vi "ShooterHoodPositionControl.vi"(0 "ShooterHoodMotorControlDevRef":T1={"DeviceStatus"={"status"=FALSE, "code"=0, "source"=""}, "Type"=enum."PWM", "PWM"={"PWM Channel"=enum."PWM 1", "DeadBand"={"Name"="", "maxPositivePwm"=0, "minPositivePwm"=0, "centerPwm"=0, "maxNegativePwm"=0, "minNegativePwm"=0, "angularRange"=0}}, "CAN"={"Device Number"=0, "SetOutput VI Ref"=variant(enum8{"Percent VBus", "Current", "Speed", "Position", "Voltage"} enum."Percent VBus"), "GetOutput VI Ref"=variant(refnum<k1> refnum), "Enable VI Ref"=variant(dbl 12.0), "Disable VI Ref"=variant(enum8{"Percent VBus", "Speed", "Position", "Slave", "Unchanged / Invalid", "Voltage Compensation", "Current", "Motion Profile"} enum."Percent VBus"), "Data"=variant}, "Invert"=FALSE, "DIO PWM"={"PWM \"Enable\" Channel"=enum."Invalid", "DIOChannel"=enum."Invalid", "PWM Rate"=0.0}}, 1 "Activate Auto":bool, 2 "MotorConfig":T6={"CAN Address"=0, "Invert"=FALSE, "InvertSensor"=FALSE, "Unit Conversion Factor"=0.0, "Brake Mode"=enum."Override to Brake", "Reverse Limt Switch Mode"=enum."Disabled", "Forward Limt Swith Mode"=enum."Disabled", "PWM Channel"=enum."Invalid", "Motor Controller Type"=enum."Talon SRX", "Peak Current (A)"=0, "Continuous Current (A)"=0, "Peak Duration (ms)"=0, "Current Limit Enable"=FALSE}, 3 "SetPoint(Deg)":dbl, 4 "ManualControl":dbl min=0.0 max=1.0) -> (5 "Manual?":bool, 6 "Current Position (Deg)":dbl)   [LabVIEW 2019]
uses:
  <vilib>/Rock Robotics/WPI/ThirdParty/Phoenix-LabVIEW/Motor Controller/Controls/CTRE_Phoenix_MotorControl_ControlMode.ctl
  ArgosLib/Config/ConfigComponents/TypeDefs/Config_PIDParams.ctl
  ArgosLib/ArgosLib.lvlib
  <vilib>/Rock Robotics/WPI/ThirdParty/Phoenix-LabVIEW/Motor Controller/Get/CTRE_Phoenix_MotorController_GetSelectedSensorData.vi
  <vilib>/Rock Robotics/WPI/ThirdParty/Phoenix-LabVIEW/Motor Controller/Controls/CTRE_Phoenix_MotorControl_NeutralMode.ctl
  <vilib>/Rock Robotics/WPI/ThirdParty/Phoenix-LabVIEW/Motor Controller/Controls/CTRE_Phoenix_MotorControl_LimitSwitchNormal.ctl
  <vilib>/Rock Robotics/SystemInterfaces/DIO/FPGA_DIOPWMChannel.ctl
  ArgosLib/Config/ConfigComponents/TypeDefs/Config_MotorCtrlType.ctl
  ArgosLib/Config/ConfigComponents/TypeDefs/Config_Motor.ctl
  <vilib>/Rock Robotics/WPI/PWM/WPI_PWMDeadband.ctl
  <vilib>/Rock Robotics/WPI/MotorControl/WPI_MotorControlType.ctl
  <vilib>/Rock Robotics/SystemInterfaces/DIO/FPGA_DIOChannel.ctl
  <vilib>/Rock Robotics/WPI/MotorControl/WPI_MotorControlDeviceRef.ctl
panel:
  in  "PIDParams":T10
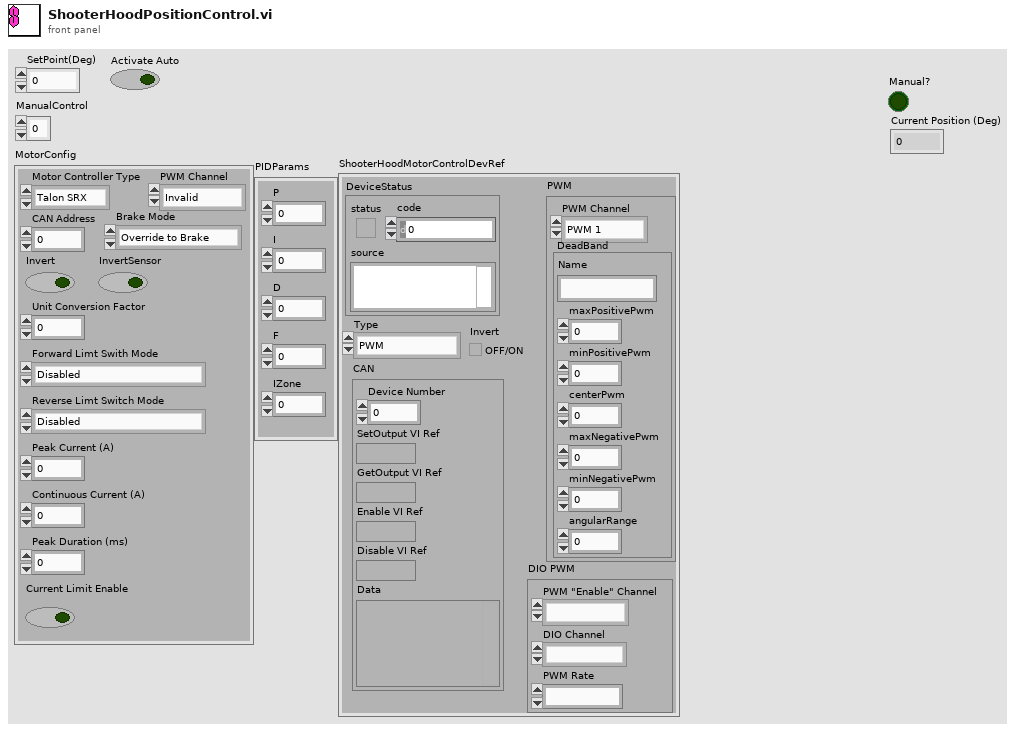
[diagram p1: front panel]
types:
  T1 = typedef "WPI_MotorControlDeviceRef.ctl" = cluster{"DeviceStatus":errorcluster, "Type":T2, "PWM":cluster{"PWM Channel":T3, "DeadBand":T4}, "CAN":cluster{"Device Number":u8, "SetOutput VI Ref":variant, "GetOutput VI Ref":variant, "Enable VI Ref":variant, "Disable VI Ref":variant, "Data":variant}, "Invert":bool, "DIO PWM":cluster{"PWM \"Enable\" Channel":T3, "DIOChannel":T5, "PWM Rate":dbl}}
  T2 = typedef "WPI_MotorControlType.ctl" = enum16{"PWM", "CAN", "DIO PWM"}
  T3 = typedef "FPGA_DIOPWMChannel.ctl" = enum8{"PWM 0", "PWM 1", "PWM 2", "PWM 3", "PWM 4", "PWM 5", "PWM 6", "PWM 7", "PWM 8", "PWM 9", "PWM MXP 0", "PWM MXP 1", "PWM MXP 2", "PWM MXP 3", "PWM MXP 4", "PWM MXP 5", "PWM MXP 6", "PWM MXP 7", "PWM MXP 8", "PWM MXP 9", "Invalid"}
  T4 = typedef "WPI_PWMDeadband.ctl" = cluster{"Name":string, "maxPositivePwm":i32, "minPositivePwm":i32, "centerPwm":i32, "maxNegativePwm":i32, "minNegativePwm":i32, "angularRange":u16}
  T5 = typedef "FPGA_DIOChannel.ctl" = enum8{"DIO 0", "DIO 1", "DIO 2", "DIO 3", "DIO 4", "DIO 5", "DIO 6", "DIO 7", "DIO 8", "DIO 9", "DIO MXP 0", "DIO MXP 1", "DIO MXP 2", "DIO MXP 3", "DIO MXP 4", "DIO MXP 5", "DIO MXP 6", "DIO MXP 7", "DIO MXP 8", "DIO MXP 9", "DIO MXP 10", "DIO MXP 11", "DIO MXP 12", "DIO MXP 13", "DIO MXP 14", "DIO MXP 15", "SPI Port CS1", "SPI Port CS2", "SPI Port CS3", "SPI Port MISO", "SPI Port MOSI", "Invalid"}
  T6 = typedef "ArgosLib.lvlib/Config_Motor.ctl" = cluster{"CAN Address":u8, "Invert":bool, "InvertSensor":bool, "Unit Conversion Factor":dbl, "Brake Mode":T7, "Reverse Limt Switch Mode":T8, "Forward Limt Swith Mode":T8, "PWM Channel":T3, "Motor Controller Type":T9, "Peak Current (A)":i32, "Continuous Current (A)":i32, "Peak Duration (ms)":i32, "Current Limit Enable":bool}
  T7 = typedef "CTRE_Phoenix_MotorControl_NeutralMode.ctl" = enum8{"EEPROMSetting", "Override to Coast", "Override to Brake"}
  T8 = typedef "CTRE_Phoenix_MotorControl_LimitSwitchNormal.ctl" = enum16{"Normally Open", "Normally Closed", "Disabled"}
  T9 = typedef "ArgosLib.lvlib/Config_MotorCtrlType.ctl" = enum16{"Disabled", "Talon SRX", "Talon SR", "Venom", "Spark MAX"}
  T10 = typedef "ArgosLib.lvlib/Config_PIDParams.ctl" = cluster{"P":dbl, "I":dbl, "D":dbl, "F":dbl, "IZone":dbl}
  T11 = cluster{"P":bool, "I":bool, "D":bool, "F":bool, "IZone":bool}
  T12 = typedef "CTRE_Phoenix_MotorControl_ControlMode.ctl" = u16
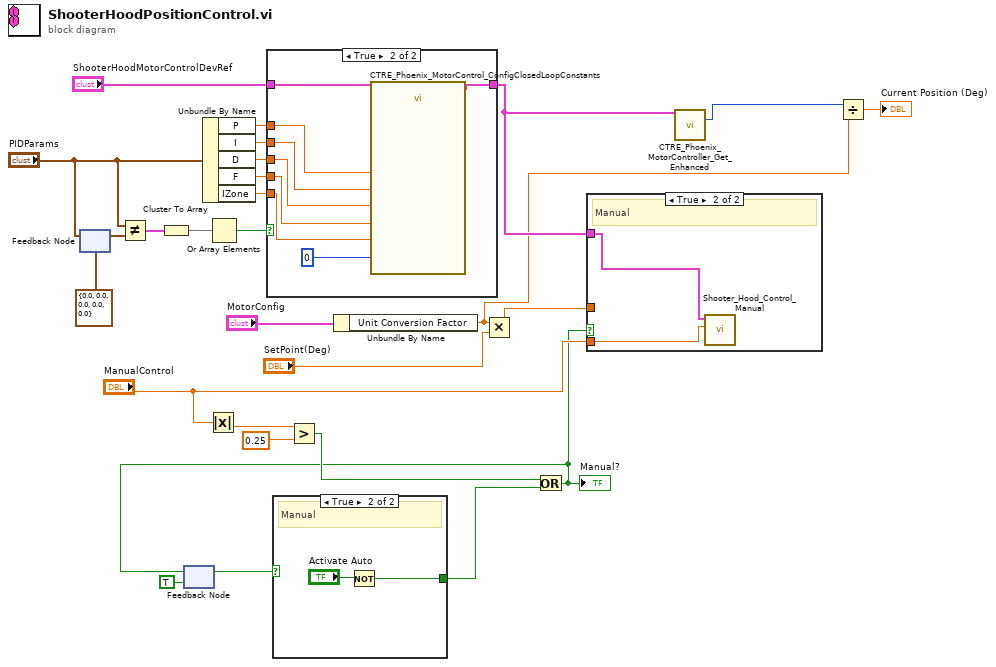
[diagram p0: block diagram]
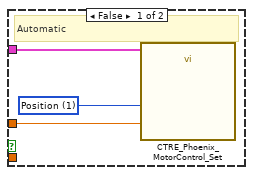
[diagram p3: hidden frame]
diagram:
  n1 = feedback-in #1("PIDParams") -> ()
  n2 = feedback #1(T10 {"P"=0.0, "I"=0.0, "D"=0.0, "F"=0.0, "IZone"=0.0} ("PIDParams")) -> (w25:T10)
  n3 = Not Equal?(x="PIDParams", y=w25) -> (x != y?=w24:T11)
  n4 = Cluster To Array(cluster=w24) -> (array=w23:bool[])
  n5 = feedback #2(TRUE) -> (w10:bool)
  n6 = Unbundle By Name("PIDParams") -> ("P"=w19:dbl, "I"=w18:dbl, "D"=w17:dbl, "F"=w16:dbl, "IZone"=w15:dbl)
  n7 = Absolute Value(x="ManualControl") -> (abs(x)=w11:dbl)
  n8 = Or Array Elements(Boolean array=w23) -> (logical OR=w21:bool)
  n9 = case shown="True" w21 {
    tunnel: "ShooterHoodMotorControlDevRef" -> [w28 w36]
    tunnel: w19 -> [_ w33]
    tunnel: w18 -> [_ w32]
    tunnel: w17 -> [_ w31]
    tunnel: w16 -> [_ w30]
    tunnel: w15 -> [_ w29]
    tunnel: [w28 w35] -> w4
    frame False {
    }
    frame True {
      n10 = call <vilib>:"CTRE_Phoenix_MotorControl_ConfigClosedLoopConstants.vi"("PhoenixMotorControlDevRef"=w36, "slotIdx"=0, "P"=w33, "I"=w32, "D"=w31, "F"=w30, "I Zone"=w29) -> ("PhoenixMotorControlDevRef"=w35:T1)  [unwired: 7 in, 1 out]
    }
  }
  n11 = case shown="True" w10 {
    selector: w10 -> [w37 _]
    tunnel: [w37 w38] -> w9
    frame False {
      # "Automatic"
    }
    frame True {
      # "Manual"
      n12 = Not(x="Activate Auto") -> (.not. x?=w38:bool)
    }
  }
  n13 = Greater?(x=w11, y=0.25) -> (0:w8:bool)
  n14 = Unbundle By Name("MotorConfig") -> ("Unit Conversion Factor"=w2:dbl)
  n15 = Multiply(x=w2, y="SetPoint(Deg)") -> (x*y=w13:dbl)
  n16 = Or(x=w8, y=w9) -> (x .or. y?=w6:bool)
  "Manual?" <- w6
  n17 = feedback-in #2(w6) -> ()
  n18 = case shown="True" w6 {
    tunnel: w13 -> [w42 _]
    tunnel: w4 -> [w41 w43]
    tunnel: "ManualControl" -> [_ w44]
    frame False {
      w40 = T12 1 items=["PercentOutput"=0, "Position"=1, "Velocity"=2, "Current"=3, "Follower"=5, "MotionProfile"=6, "MotionMagic"=7, "MotionProfileArc"=10, "Disabled"=15] ("Control Mode")
      # "Automatic"
      n19 = call <vilib>:"CTRE_Phoenix_MotorControl_Set.vi"("Output"=w42, "Control Mode"=w40, "PhoenixMotorControlDevRef"=w41) -> ()  [unwired: 7 in, 2 out]
    }
    frame True {
      # "Manual"
      n20 = call "Shooter_Hood_Control_Manual.vi"("Hood_Command"=w44, "Shooter_Hood_DevRef"=w43) -> ()  [unwired: 10 in]
    }
  }
  n21 = call-poly <vilib>:"CTRE_Phoenix_MotorController_Get_Enhanced.vi"("PhoenixMotorControlDevRef"=w4) -> ("Position (Raw Sensor Units)"=w3:i32)  [unwired: 11 in, 3 out]
  n22 = Divide(x=w3, y=w2) -> (x/y=→"Current Position (Deg)":dbl)
